vi "Launcher Discover.vi"(6 "contextId":T1, 8 "error in":errorcluster, 9 "timeout (ms)":i32=-1, 10 "Request Data":T7, 11 "gRPC ID":T1) -> (0 "error out":errorcluster, 2 "Response Data":T2, 3 "gRPC ID out":T1)   [LabVIEW 2021, in "CIF_Launcher_client.lvlib"]
uses:
  CIF_Launcher_client.lvlib
  <vilib>/gRPC/LabVIEW gRPC Library/Shared/grpcId.ctl
  RPC Messages/cif_launcher_DiscoverCommand.ctl
  RPC Messages/cif_launcher_DiscoveredPlugins.ctl
  RPC Messages/cif_launcher_DiscoveredPlugin.ctl
  RPC Messages/cif_common_Version.ctl
  RPC Messages/cif_manager_PluginMetadata.ctl
  RPC Messages/cif_common_Status.ctl
  RPC Messages/cif_launcher_DiscoveredPlugins_Flat.ctl
  RPC Messages/cif_launcher_DiscoveredPlugin_Flat.ctl
  RPC Messages/cif_common_Version_Flat.ctl
  RPC Messages/cif_manager_PluginMetadata_Flat.ctl
  RPC Messages/cif_common_Status_Flat.ctl
  14035477-4c25-4107-8ed5-d0c4ef420ce5.vi
  <vilib>/gRPC/LabVIEW gRPC Library/Shared/TranslateGrpcError.vi
  <vilib>/gRPC/LabVIEW gRPC Library/Shared/Wait On Occurrence Wrapper.vi
  RPC Messages/FlatToRichcif_launcher_DiscoveredPlugin.vi
  RPC Messages/FlatToRichcif_common_Status.vi
  <vilib>/gRPC/LabVIEW gRPC Library/Shared/Wait On Occurence.vi
  RPC Messages/FlatToRichcif_common_Version.vi
  RPC Messages/FlatToRichcif_manager_PluginMetadata.vi
  <vilib>/gRPC/LabVIEW gRPC Library/Server API/Server/Get Server DLL Path.vi
  <vilib>/Utility/error.llb/Error Cluster From Error Code.vi
  <vilib>/Utility/config.llb/Open Config Data.vi
  <vilib>/Utility/config.llb/Write Key.vi
  <vilib>/Utility/config.llb/Write Key (Boolean).vi
  <vilib>/Utility/config.llb/Not A Config Data Refnum.vi
  <vilib>/Utility/config.llb/Read Key.vi
  <vilib>/Utility/config.llb/Read Key (Boolean).vi
  <vilib>/Utility/config.llb/Close Config Data.vi
  <vilib>/gRPC/LabVIEW gRPC Library/grpc-lvsupport-release.lvlib
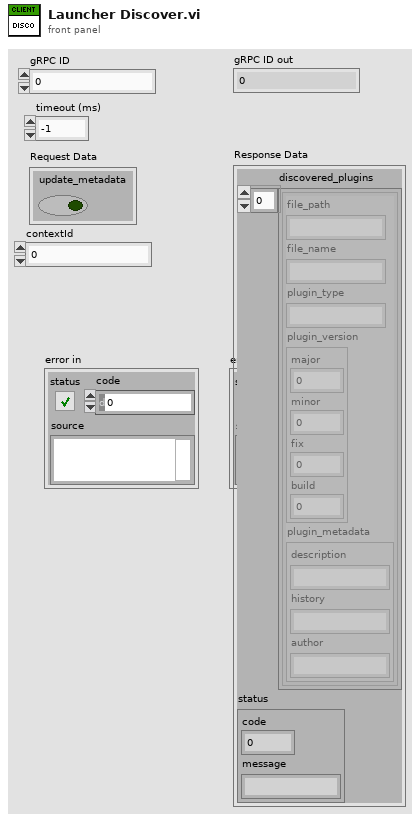
[diagram p1: front panel]
types:
  T1 = typedef "grpc-lvsupport-release.lvlib/grpcId.ctl" = u64
  T2 = typedef "CIF_Launcher_client.lvlib/cif_launcher_DiscoveredPlugins.ctl" = cluster{"discovered_plugins":T3[], "status":T6}
  T3 = typedef "CIF_Launcher_client.lvlib/cif_launcher_DiscoveredPlugin.ctl" = cluster{"file_path":string, "file_name":string, "plugin_type":string, "plugin_version":T4, "plugin_metadata":T5}
  T4 = typedef "CIF_Launcher_client.lvlib/cif_common_Version.ctl" = cluster{"major":u32, "minor":u32, "fix":u32, "build":u32}
  T5 = typedef "CIF_Launcher_client.lvlib/cif_manager_PluginMetadata.ctl" = cluster{"description":string, "history":string, "author":string}
  T6 = typedef "CIF_Launcher_client.lvlib/cif_common_Status.ctl" = cluster{"code":i32, "message":string}
  T7 = typedef "CIF_Launcher_client.lvlib/cif_launcher_DiscoverCommand.ctl" = cluster{"update_metadata":bool}
  T8 = typedef "CIF_Launcher_client.lvlib/cif_launcher_DiscoveredPlugins_Flat.ctl" = cluster{"discovered_plugins":T9[], "status":T12}
  T9 = typedef "CIF_Launcher_client.lvlib/cif_launcher_DiscoveredPlugin_Flat.ctl" = cluster{"file_path":string, "file_name":string, "plugin_type":string, "plugin_version":T10, "plugin_metadata":T11}
  T10 = typedef "CIF_Launcher_client.lvlib/cif_common_Version_Flat.ctl" = cluster{"major":u32, "minor":u32, "fix":u32, "build":u32}
  T11 = typedef "CIF_Launcher_client.lvlib/cif_manager_PluginMetadata_Flat.ctl" = cluster{"description":string, "history":string, "author":string}
  T12 = typedef "CIF_Launcher_client.lvlib/cif_common_Status_Flat.ctl" = cluster{"code":i32, "message":string}
  T13 = typedef "CIF_Launcher_client.lvlib/cif_launcher_DiscoverCommand_Flat.ctl" = cluster{"update_metadata":bool}
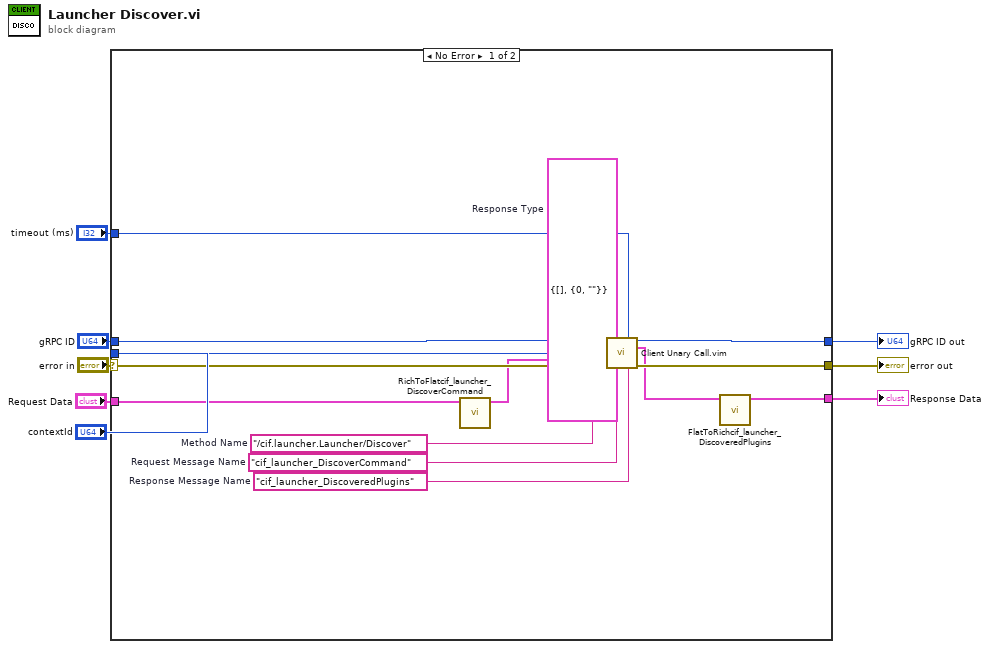
[diagram p0: block diagram]
diagram:
  n1 = case shown="No Error" "error in" {
    selector: "error in" -> [w18 w23]
    tunnel: [w17 w23] -> w7
    tunnel: "gRPC ID" -> [w16 w24]
    tunnel: [w15 w24] -> w5
    tunnel: "Request Data" -> [w12 _]
    tunnel: [w9 _] -> w3
    tunnel: "timeout (ms)" -> [w14 _]
    tunnel: "contextId" -> [w13 _]
    frame No Error {
      w19 = "cif_launcher_DiscoveredPlugins"  # Response Message Name
      w20 = "cif_launcher_DiscoverCommand"  # Request Message Name
      w21 = T8 {"discovered_plugins"=[], "status"={"code"=0, "message"=""}}  # Response Type
      w22 = "/cif.launcher.Launcher/Discover"  # Method Name
      n2 = call "RichToFlatcif_launcher_DiscoverCommand.vi"("InputCluster"=w12) -> ("OutputCluster"=w11:T13)  [unwired: 10 in]
      n3 = call "Client Unary Call.vim"("ClientID in"=w16, "Response Type"=w21, "timeout (ms)"=w14, "Method Name"=w22, "contextId"=w13, "Request Data"=w11, "error in"=w18, "Request Message Name"=w20, "Response Message Name"=w19) -> ("ClientID out"=w15:u64, "Response Data"=w10:T8, "error out"=w17:errorcluster)  [unwired: 4 in]
      n4 = call "FlatToRichcif_launcher_DiscoveredPlugins.vi"("InputCluster"=w10) -> ("OutputCluster"=w9:T2)  [unwired: 10 in]
    }
    frame Error {
    }
  }
  "error out" <- w7
  "gRPC ID out" <- w5
  "Response Data" <- w3
